vi "niScope Multi Fetch Cluster Complex Double.vi"(7 "timeout":dbl=5.0 format="%.2f", 8 "error in":errorcluster, 9 "numSamples":i32=-1, 10 "channels":string="0", 11 "instrument handle":refnum<k15>) -> (0 "error out":errorcluster, 1 "waveform":cluster{"t0":dbl, "dt":dbl, "Y":cdb[]}[](array[cluster]) {"Y" format="%.2f"; "dt" format="%.2f"; "t0" format="%.2f"}, 2 "wfm info":T1(array[cluster]) {"reserved2" format="%.2f"; "reserved1" format="%.2f"; "offset" format="%^.3e"; "gain" format="%^.3e"; "xIncrement" format="%^.3e"; "relativeInitialX" format="%^.3e"; "absoluteInitialX" format="%^.3e"}, 3 "instrument handle out":refnum<k15>)   [LabVIEW 2020]
doc: "Retrieves the waveform the digitizer has acquired for multiple channels and records. Returns a one-dimensional array of complex, scaled waveforms in clusters that include timing information."
uses:
  niScope_32.dll
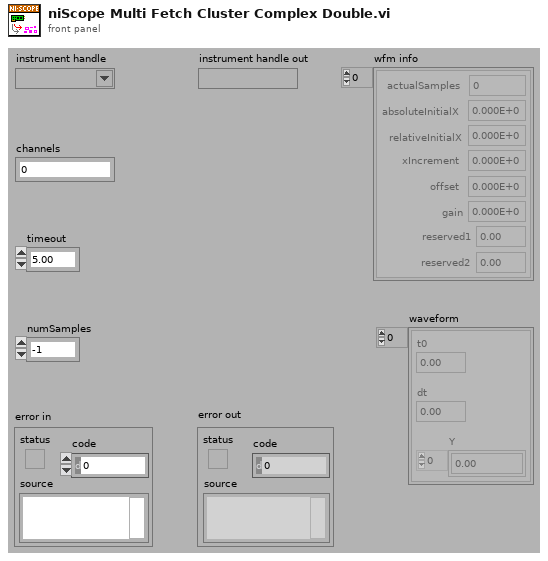
[diagram p1: front panel]
types:
  T1 = cluster{"actualSamples":i32, "absoluteInitialX":dbl, "relativeInitialX":dbl, "xIncrement":dbl, "offset":dbl, "gain":dbl, "reserved1":dbl, "reserved2":dbl}[]
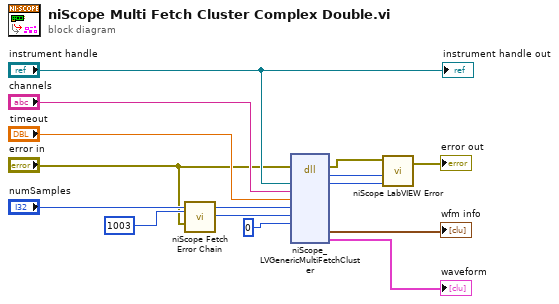
[diagram p0: block diagram]
diagram:
  n1 = call "niScope Fetch Error Chain.vi"("dataType in"=1003 ("dataType"), "error in"="error in") -> ("dataType"=w6:i32)  [unwired: 13 in]
  n2 = dll-call lib="niScope_*.*" fn="niScope_LVGenericMultiFetchCluster"(error in="error in", "instrument handle"="instrument handle", "channel"="channels", "timeout"="timeout", "numSamples"="numSamples", "dataType"=w6, "interleaved"=0 ("y")) -> (error out=w1:errorcluster, "status"=w8:i32, "instrument handle"=w7:u32, "wfm info"=→"wfm info":T1, "waveform"=→"waveform":cluster{"t0":dbl, "dt":dbl, "Y":cdb[]}[])  [unwired: 9 in, 1 out]
  n3 = call "niScope LabVIEW Error.vi"("instrument handle"=w7, "niScope error code (0)"=w8, "error in (no error)"=w1) -> ("error out"=→"error out":errorcluster)  [unwired: 2 in]
  "instrument handle out" <- "instrument handle"
